vi "test_Create MetaData Channel_error on empty name.vi"(8 "error in (no error)":errorcluster, 11 "TestCase in":refnum<class "Instrument Addon Scripting API Channels Unit Tests.lvclass">) -> (0 "error out":errorcluster, 3 "TestCase out":refnum<class "Instrument Addon Scripting API Channels Unit Tests.lvclass">)   [LabVIEW 2019, in "Instrument Addon Scripting API Channels Unit Tests.lvclass"]
uses:
  Instrument Addon Scripting API Channels Unit Tests.lvclass
  APIs/Scripting API/TypeDefs/Single Channel Format Settings.ctl
  Instrument Addon Scripting API Channels Unit Tests.lvclass/Instrument Addon Scripting API Channels Unit Tests.ctl
  <vilib>/NI VeriStand/Custom Device Tools/Custom Device Utility Library/NI VeriStand - Search for Item by Name.vi
  APIs/Scripting API/Channels/Create MetaData Channel - Single Channel - Format.vi
  <vilib>/addons/_JKI Toolkits/VI Tester/TestCase.llb/TestCase.lvclass
  Instrument Addon Scripting API Test Assets/Instrument Addon Scripting API Test Assets.lvclass
  <vilib>/NI VeriStand/Custom Device Tools/Custom Device Utility Library/Custom Device Utility Library.lvlib
  APIs/Scripting API/Instrument Addon Scripting API.lvlib
  C:/Program Files (x86)/National Instruments/LabVIEW 2019/vi.lib/addons/_JKI Toolkits/VI Tester/TestCase.llb/TestCase.lvclass
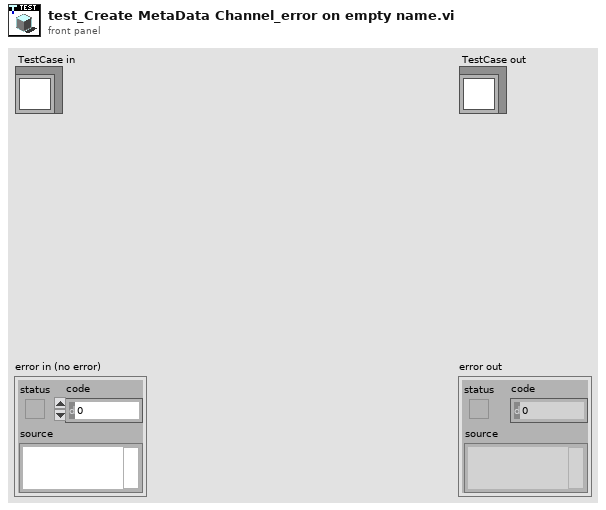
[diagram p1: front panel]
types:
  T1 = typedef "Instrument Addon Scripting API.lvlib/Single Channel Format Settings.ctl" = cluster{"Format String":string, "Default Value":dbl, "Units":string}
  T2 = typedef "Custom Device API.lvlib/Custom Device Item Ref.ctl" = u64
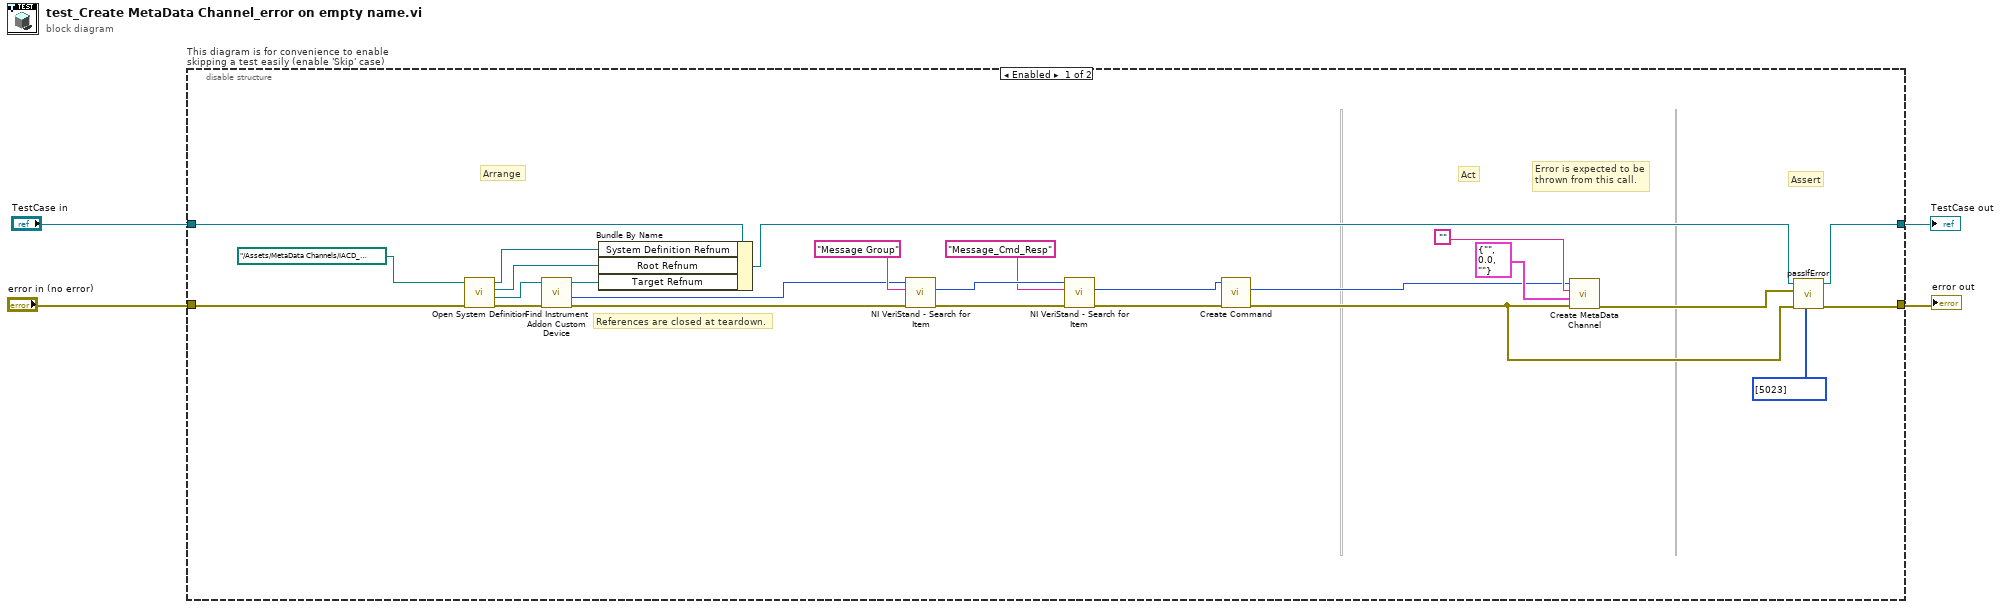
[diagram p0: block diagram]
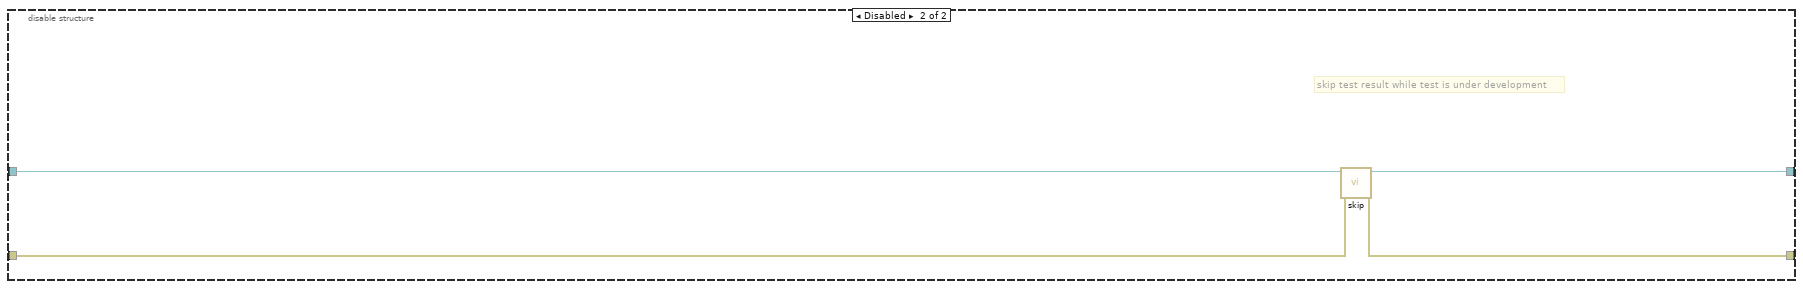
[diagram p2: hidden frame]
diagram:
  n1 = disable-structure "This diagram is for convenience to enable skipping a test easily (enable 'Skip' case)" shown="Enabled" {
    disable-tunnel: "TestCase in" -> [w21 w33]
    disable-tunnel: [w26 w31] -> w1
    disable-tunnel: [w25 w32] -> w3
    disable-tunnel: "error in (no error)" -> [w29 w30]
    frame Enabled {
      # "Error is expected to be\nthrown from this call."
      # "Assert"
      # "References are closed at teardown."
      # "Act"
      # "Arrange"
      n2 = call "Open System Definition.vi"("error in (no error)"=w29, "System Definition File"=path "../Assets/MetaData Channels/IACD_channels.nivssdf") -> ("error out"=w27:errorcluster, "Target Refnum"=w28:refnum<k24>, "Root Refnum"=w23:refnum<k24>, "System Definition Refnum"=w22:refnum<k24>)  [unwired: 6 in]
      n3 = call "Find Instrument Addon Custom Device.vi"("error in"=w27, "target in"=w28) -> ("error out"=w16:errorcluster, "NodeID"=w15:u64, "target out"=w24:refnum<k24>)  [unwired: 7 in]
      n4 = Bundle By Name(cluster=w21, "System Definition Refnum"=w22, "Root Refnum"=w23, "Target Refnum"=w24) -> (w14:refnum<class "Instrument Addon Scripting API Channels Unit Tests.lvclass">)
      n5 = call-poly <vilib>:"NI VeriStand - Search for Item.vi"("error in"=w16, "Item Name"="Message Group", "Section Ref in"=w15) -> ("error out"=w17:errorcluster, "Item Ref"=w19:T2)  [unwired: 5 in, 2 out]
      n6 = call-poly <vilib>:"NI VeriStand - Search for Item.vi"("error in"=w17, "Item Name"="Message_Cmd_Resp", "Section Ref in"=w19) -> ("error out"=w8:errorcluster, "Item Ref"=w5:T2)  [unwired: 5 in, 2 out]
      n7 = call "Create Command.vi"("error in"=w8, "message refnum In"=w5) -> ("error out"=w7:errorcluster, "command refnum"=w6:T2)  [unwired: 7 in, 1 out]
      n8 = call-poly "Create MetaData Channel.vi"("error in (no error)"=w7, "settings"=T1 {"Format String"="", "Default Value"=0.0, "Units"=""} ("Settings"), "channel name"="", "command refnum in"=w6) -> ("error out"=w11:errorcluster)  [unwired: 5 in, 2 out]
      n9 = call-dynamic "passIfError.vi"("passing error codes (default = any error code)"=i32[] [5023], "error in (no error)"=w7, "error"=w11, "TestCase in"=w14) -> ("error out"=w25:errorcluster, "TestCase out"=w26:refnum<class "Instrument Addon Scripting API Channels Unit Tests.lvclass">)  [unwired: 6 in]
    }
    frame Disabled {
      # "skip test result while test is under development"
      n10 = call <vilib>:"skip.vi"("error in (no error)"=w30, "TestCase in"=w33) -> ("error out"=w32:errorcluster, "TestCase out"=w31:refnum<class "Instrument Addon Scripting API Channels Unit Tests.lvclass">)  [unwired: 8 in]
    }
  }
  "error out" <- w3
  "TestCase out" <- w1
